vi "Calculate X Bar.vi"(11 "2D Array In":dbl[][](array[numeric])) -> (1 "Xbar":dbl format="%0.6f", 2 "Average Array":dbl[](array[numeric]), 3 "2D Array Out":dbl[][](array[numeric]))   [LabVIEW 2018, in "GRR Core.lvclass"]
uses:
  GRR Core.lvclass
  <vilib>/Analysis/baseanly.llb/Mean (DBL).vi
  <vilib>/Analysis/NI_AALBase.lvlib
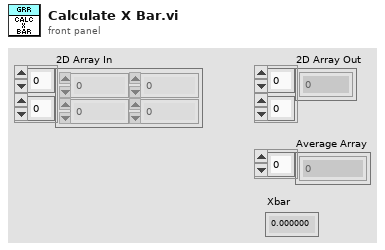
[diagram p1: front panel]
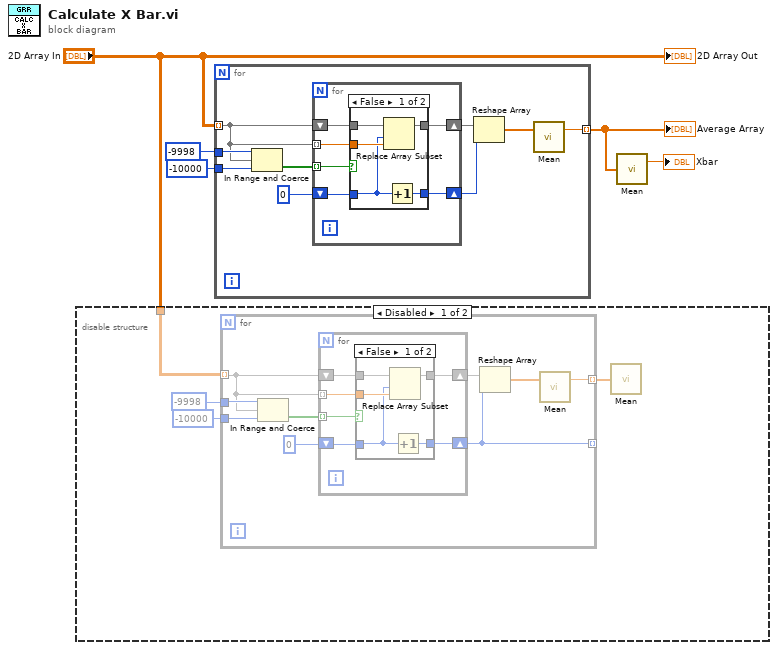
[diagram p0: block diagram]
diagram:
  n1 = disable-structure shown="Disabled" {
    disable-tunnel: "2D Array In" -> [w6 _]
    frame Disabled {
      n2 = for {
        tunnel: [w18] -> w7 mode=indexing
        tunnel: -9998 -> [w17]
        tunnel: -10000 -> [w16]
        tunnel: [w11] -> _ mode=indexing
        tunnel: w6 -> [w10] mode=indexing
        n3 = In Range and Coerce(upper limit=w17, x=w10, lower limit=w16) -> (In Range?=w14:bool[])  [unwired: 1 out]
        n4 = for {
          shift-right: [w24] -> w15
          shift-left: w10 -> [w23]
          tunnel: w14 -> [w22] mode=indexing
          tunnel: w10 -> [w21] mode=indexing
          shift-right: [w19] -> w11
          shift-left: 0 -> [w20]
          n5 = case shown="False" w22 {
            tunnel: [w29 w30] -> w24
            tunnel: w23 -> [w28 w30]
            tunnel: w21 -> [w27 _]
            tunnel: w20 -> [w26 w31]
            tunnel: [w25 w31] -> w19
            frame False {
              n6 = Replace Array Subset(array=w28, new element=w27, index=w26) -> (w29:dbl[])
              n7 = Increment(x=w26) -> (x+1=w25:i32)
            }
            frame True {
            }
          }
        }
        n8 = Reshape Array(w15, w11) -> (w12:dbl[])
        n9 = call-poly <vilib>:"Mean.vi"("X"=w12) -> ("mean"=w18:dbl)  [unwired: 1 out]
      }
      n10 = call-poly <vilib>:"Mean.vi"("X"=w7) -> ()  [unwired: 2 out]
    }
    frame Enabled {
    }
  }
  n11 = for {
    tunnel: "2D Array In" -> [w35] mode=indexing
    tunnel: [w40] -> w2 mode=indexing
    tunnel: -9998 -> [w39]
    tunnel: -10000 -> [w38]
    n12 = In Range and Coerce(upper limit=w39, x=w35, lower limit=w38) -> (In Range?=w36:bool[])  [unwired: 1 out]
    n13 = for {
      shift-right: [w46] -> w37
      shift-left: w35 -> [w45]
      tunnel: w36 -> [w44] mode=indexing
      tunnel: w35 -> [w43] mode=indexing
      shift-right: [w41] -> w32
      shift-left: 0 -> [w42]
      n14 = case shown="False" w44 {
        tunnel: [w51 w52] -> w46
        tunnel: w45 -> [w50 w52]
        tunnel: w43 -> [w49 _]
        tunnel: w42 -> [w48 w53]
        tunnel: [w47 w53] -> w41
        frame False {
          n15 = Replace Array Subset(array=w50, new element=w49, index=w48) -> (w51:dbl[])
          n16 = Increment(x=w48) -> (x+1=w47:i32)
        }
        frame True {
        }
      }
    }
    n17 = Reshape Array(w37, w32) -> (w33:dbl[])
    n18 = call-poly <vilib>:"Mean.vi"("X"=w33) -> ("mean"=w40:dbl)  [unwired: 1 out]
  }
  "Average Array" <- w2
  n19 = call-poly <vilib>:"Mean.vi"("X"=w2) -> ("mean"=→"Xbar":dbl)  [unwired: 1 out]
  "2D Array Out" <- "2D Array In"
